vi "Config_Image_Read.vi"(8 "error in (no error)":errorcluster) -> (0 "error out":errorcluster)   [LabVIEW 2020]
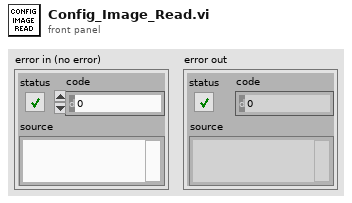
[diagram p1: front panel]
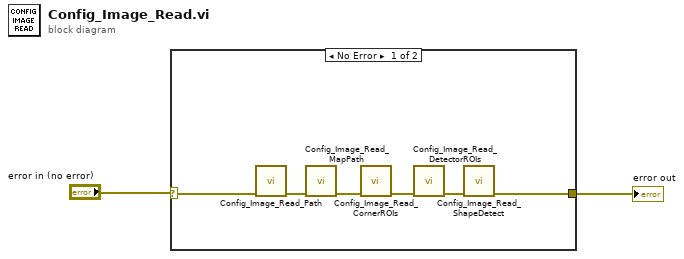
[diagram p0: block diagram]
diagram:
  n1 = case shown="No Error" "error in (no error)" {
    selector: "error in (no error)" -> [w8 w9]
    tunnel: [w5 w9] -> w1
    frame No Error {
      n2 = call "Config_Image_Read_Path.vi"("error in (no error)"=w8) -> ("error out"=w4:errorcluster)  [unwired: 10 in]
      n3 = call "Config_Image_Read_MapPath.vi"("error in (no error)"=w4) -> ("error out"=w3:errorcluster)  [unwired: 10 in]
      n4 = call "Config_Image_Read_CornerROIs.vi"("error in (no error)"=w3) -> ("error out"=w7:errorcluster)  [unwired: 10 in]
      n5 = call "Config_Image_Read_DetectorROIs.vi"("error in (no error)"=w7) -> ("error out"=w6:errorcluster)  [unwired: 10 in]
      n6 = call "Config_Image_Read_ShapeDetect.vi"("error in (no error)"=w6) -> ("error out"=w5:errorcluster)  [unwired: 10 in]
    }
    frame Error {
    }
  }
  "error out" <- w1
